vi "Agilent DMM Config Test.vi"(8 "error in (no error)":errorcluster, 10 "Configuration":T1={"BusType"=enum."GPIB", "GPIB Bus"=0, "GPIB Address"=16, "IP"=0, "COM"=1, "Baud Rate"=enum."9600"}, 11 "Str Refnum":refnum<vi>) -> (0 "error out":errorcluster, 3 "Serial Number":string)   [LabVIEW 2011]
uses:
  TypeDefs/Agilent DMM Configuration.ctl
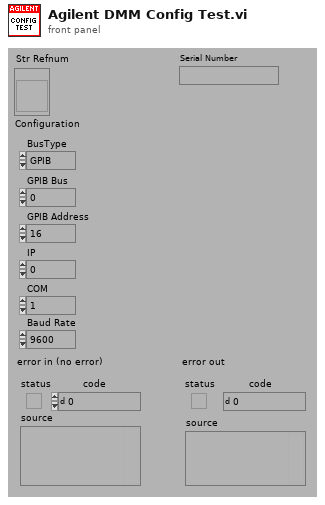
[diagram p1: front panel]
types:
  T1 = typedef "Agilent DMM Configuration.ctl" = cluster{"BusType":enum32{"GPIB", "LAN/IP", "Serial"}, "GPIB Bus":i32, "GPIB Address":i32, "IP":u32, "COM":i32, "Baud Rate":enum16{"300", "600", "1200", "2400", "4800", "9600"}}
  T2 = typedef "Agilent DMM Instrument Info.ctl" = cluster{"Model":string, "Serial":string, "Firmware":string}
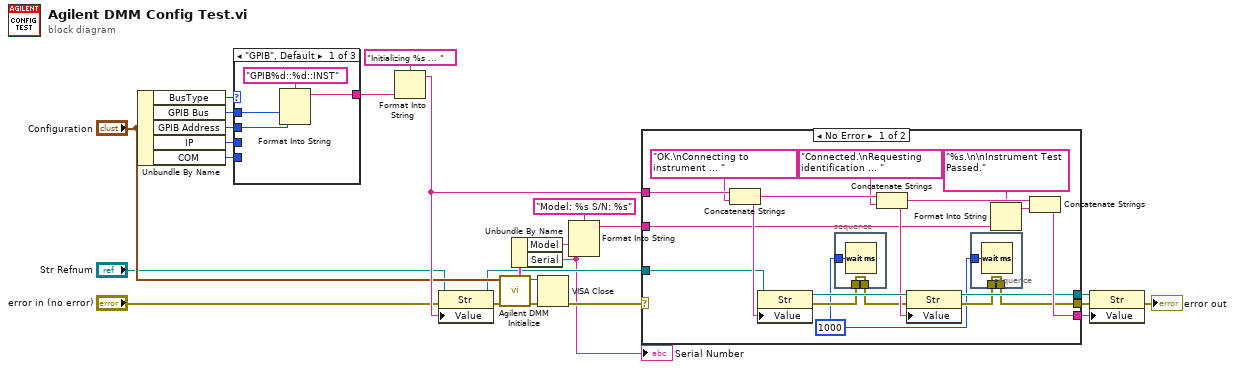
[diagram p0: block diagram]
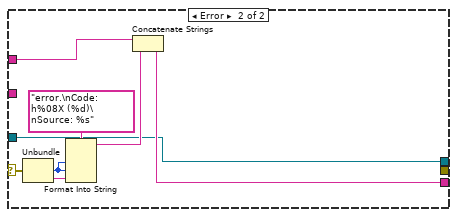
[diagram p2: hidden frame]
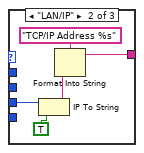
[diagram p3: hidden frame]
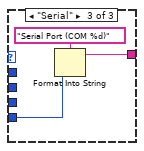
[diagram p4: hidden frame]
diagram:
  n1 = Unbundle By Name("Configuration") -> ("BusType"=w24:enum32{"GPIB", "LAN/IP", "Serial"}, "GPIB Bus"=w23:i32, "GPIB Address"=w22:i32, "IP"=w21:u32, "COM"=w20:i32)
  n2 = case shown="\"GPIB\", Default" w24 {
    tunnel: w23 -> [w28 _ _]
    tunnel: w22 -> [w27 _ _]
    tunnel: w21 -> [_ w33 _]
    tunnel: w20 -> [_ _ w36]
    tunnel: [w26 w30 w35] -> w19
    frame "GPIB", Default {
      n3 = Format Into String(format string="GPIB%d::%d::INST", w28, w27) -> (resulting string=w26:string)  [unwired: 2 in, 1 out]
    }
    frame "LAN/IP" {
      n4 = IP To String(1:TRUE, 2:w33) -> (0:w32:string)
      n5 = Format Into String(format string="TCP/IP Address %s", w32) -> (resulting string=w30:string)  [unwired: 2 in, 1 out]
    }
    frame "Serial" {
      n6 = Format Into String(format string="Serial Port (COM %d)", w36) -> (resulting string=w35:string)  [unwired: 2 in, 1 out]
    }
  }
  n7 = Format Into String(format string="Initializing %s ... ", w19) -> (resulting string=w18:string)  [unwired: 2 in, 1 out]
  n8 = property class="Str"(reference="Str Refnum", error in="error in (no error)", "Value"=w18) -> (reference out=w2:refnum<vi>, error out=w16:errorcluster)
  n9 = call "Agilent DMM Initialize.vi"("error in (no error)"=w16, "Configuration"="Configuration") -> ("error out"=w13:errorcluster, "VISA Resource Name"=w11:refnum<visa-resource-name>, "Agilent DMM"=w10:T2)  [unwired: 7 out]
  n10 = Unbundle By Name(w10) -> ("Model"=w14:string, "Serial"=w1:string)
  "Serial Number" <- w1
  n11 = VISA Close(VISA resource name=w11, error in (no error)=w13) -> (error out=w12:errorcluster)
  n12 = Format Into String(format string="Model: %s S/N: %s" ("Return Model and Serial #"), w14, w1) -> (resulting string=w9:string)  [unwired: 2 in, 1 out]
  n13 = case shown="No Error" w12 {
    selector: w12 -> [_ w64]
    tunnel: w18 -> [w53 w66]
    tunnel: w2 -> [w48 w59]
    tunnel: w9 -> [w45 _]
    tunnel: [w44 w60] -> w7
    tunnel: [w43 w59] -> w5
    tunnel: [w39 _] -> w4
    frame No Error {
      w38 = u32 1000 ("milliseconds to wait")
      n14 = Concatenate Strings(w53, "OK.\nConnecting to instrument ... ") -> (w51:string)
      n15 = property class="Str"(reference=w48, "Value"=w51) -> (reference out=w54:refnum<vi>, error out=w42:errorcluster)  [unwired: 1 in]
      n16 = stacked-sequence {
        tunnel: w38 -> [w58]
        tunnel: w42 -> [w57]
        tunnel: [w57] -> w41
        frame #0 {
          n17 = Wait (ms)(milliseconds to wait=w58) -> ()  [unwired: 1 out]
        }
      }
      n18 = Concatenate Strings(w51, "Connected.\nRequesting identification ... ") -> (w49:string)
      n19 = property class="Str"(reference=w54, error in=w41, "Value"=w49) -> (reference out=w43:refnum<vi>, error out=w40:errorcluster)
      n20 = stacked-sequence {
        tunnel: w38 -> [w56]
        tunnel: w40 -> [w55]
        tunnel: [w55] -> w39
        frame #0 {
          n21 = Wait (ms)(milliseconds to wait=w56) -> ()  [unwired: 1 out]
        }
      }
      n22 = Format Into String(format string="%s.\n\nInstrument Test Passed.", w45) -> (resulting string=w46:string)  [unwired: 2 in, 1 out]
      n23 = Concatenate Strings(w49, w46) -> (w44:string)
    }
    frame Error {
      n24 = Unbundle(w64) -> ("code"=w63:i32, "source"=w62:string)  [unwired: 1 out]
      n25 = Format Into String(format string="error.\nCode:  h%08X (%d)\nSource: %s", w63, w63, w62) -> (resulting string=w61:string)  [unwired: 2 in, 1 out]
      n26 = Concatenate Strings(w66, w61) -> (w60:string)
    }
  }
  n27 = property class="Str"(reference=w5, error in=w4, "Value"=w7) -> (error out=→"error out":errorcluster)  [unwired: 1 out]
